vi "getXYThZ.vi"(10 "X, Y, ThZ Zero Offset":fxp<+/-,27,5>[](array[numeric])=[0.0, 0.0, 0.0], 11 "PosMeas_Array In":fxp<+/-,25,5>[](array[numeric])=[0.0, 0.0, 0.0, 0.0, 0.0, 0.0, 0.0, 0.0, 0.0, 0.0, 0.0, 0.0, 0.0]) -> (3 "X,Y,ThZ_out":fxp<+/-,27,5>[](array[numeric]) format="%#.21g")   [LabVIEW 2020, in "PositionMeas.lvlib"]
doc: "Returns the X, Y, ThZ measurements based on position sensor data"
uses:
  PositionMeas.lvlib
  <vilib>/Platform/TimedLoop/XDataNode/XDataNode.xnode
  <vilib>/Platform/TimedLoop/XDataNode/nitl_modes.ctl
  <vilib>/Platform/TimedLoop/XDataNode/XDNodeRunTimeDep.lvlib
  <vilib>/Platform/TimedLoop/XDataNode/wakeup.ctl
  <vilib>/Platform/TimedLoop/XDataNode/timing_clust.ctl
panel:
  # "To be completed..."
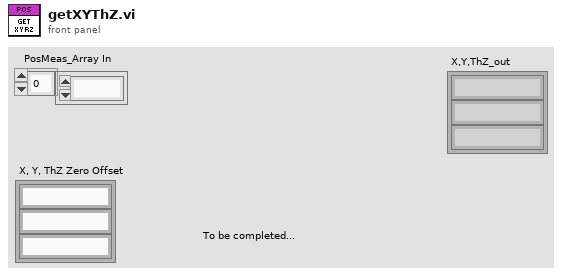
[diagram p1: front panel]
types:
  T1 = typedef "XDNodeRunTimeDep.lvlib/timing_clust.ctl" = cluster{"Expected End [f-1]":u64, "Actual End [f-1]":u64, "Finished Late? [f-1]":bool, "Expected End [i-1]":u64, "Actual End [i-1]":u64, "Finished Late? [i-1]":bool, "Expected Start [i]":u64, "Actual Start [i]":u64, "Expected Start [f]":u64, "Actual Start [f]":u64, "Source Name":string, "Structure Name":string, "Period":i64, "Deadline":i64, "Offset":i64, "Start":i64, "Priority":i32, "Timeout":i32, "Mode":T2, "Wakeup Reason":T3, "Error":errorcluster, "Source Type":string, "Secondary Source Type":string, "Global End Time":u64, "Global Start Time":u64, "Frame Duration":u64, "Iteration Duration":u64, "Assigned CPU":i32, "I/O Scan Engine Mode":u32}
  T2 = typedef "XDNodeRunTimeDep.lvlib/nitl_modes.ctl" = enum32{"No Change", "Process missed periods, maintain original phase", "Discard missed periods, maintain original phase", "Process missed periods, ignore original phase", "Discard missed periods, ignore original phase"}
  T3 = typedef "XDNodeRunTimeDep.lvlib/wakeup.ctl" = enum32{"Normal", "Aborted", "Asynchronous wakeup", "Timing source error", "Timed loop error", "Timeout"}
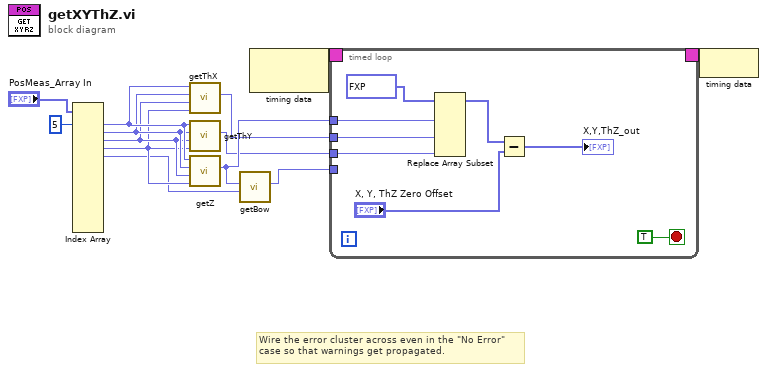
[diagram p0: block diagram]
diagram:
  # "Wire the error cluster across even in the \"No Error\"\ncase so that warnings get propagated."
  n1 = Index Array(array="PosMeas_Array In", index #1=5 ("index")) -> (element #1=w9:fxp<+/-,25,5>, element #2=w8:fxp<+/-,25,5>, element #3=w7:fxp<+/-,25,5>, element #4=w6:fxp<+/-,25,5>, element #5=w5:fxp<+/-,25,5>)  [unwired: 13 in, 9 out]
  n2 = call "getThX.vi"("SW"=w6, "NW"=w7, "NE"=w8, "SE"=w9) -> ("ThX"=w3:fxp<+/-,25,5>)  [unwired: 7 in]
  n3 = call "getThY.vi"("SW"=w6, "NW"=w7, "NE"=w8, "SE"=w9) -> ("ThY"=w2:fxp<+/-,25,5>)  [unwired: 7 in]
  n4 = call "getZ.vi"("SW"=w6, "NW"=w7, "NE"=w8, "SE"=w9) -> ("Z"=w4:fxp<+/-,25,5>)  [unwired: 7 in]
  n5 = call "getBow.vi"("CI"=w5, "Z"=w4) -> ("Bow"=w1:fxp<+/-,25,5>)  [unwired: 9 in]
  n6 = node-c288() -> (w12:T1)  [unwired: 1 in]
  n7 = timed-loop {
    timing: w12 -> [_]
    timing-out: [_] -> w11
    tunnel: w4 -> [w21]
    tunnel: w3 -> [w20]
    tunnel: w2 -> [w19]
    tunnel: w1 -> [_]
    stop <- TRUE stop-if-true
    n8 = Replace Array Subset(array=fxp<+/-,27,5>[] [0.0, 0.0, 0.0], new element #1=w21, new element #2=w20, new element #3=w19) -> (w17:fxp<+/-,27,5>[])  [unwired: 3 in]
    n9 = Subtract(x=w17, y="X, Y, ThZ Zero Offset") -> (x-y=→"X,Y,ThZ_out":fxp<+/-,27,5>[])
  }
  n10 = node-c288(w11) -> ()
